vi "demod_table.vi"(2 "Light enables":bool[](array[boolean]), 3 "Block size":i32) -> (0 "Cosine table":dbl[][][](array[numeric]) format="%#.4f", 1 "Sine table":dbl[][][](array[numeric]) format="%#.4f")   [LabVIEW 2013]
uses:
  initialization/globals.vi
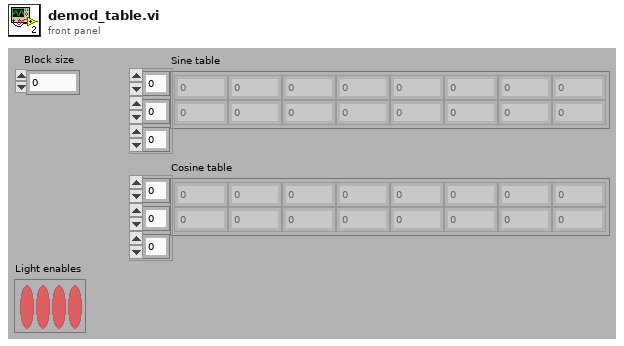
[diagram p1: front panel]
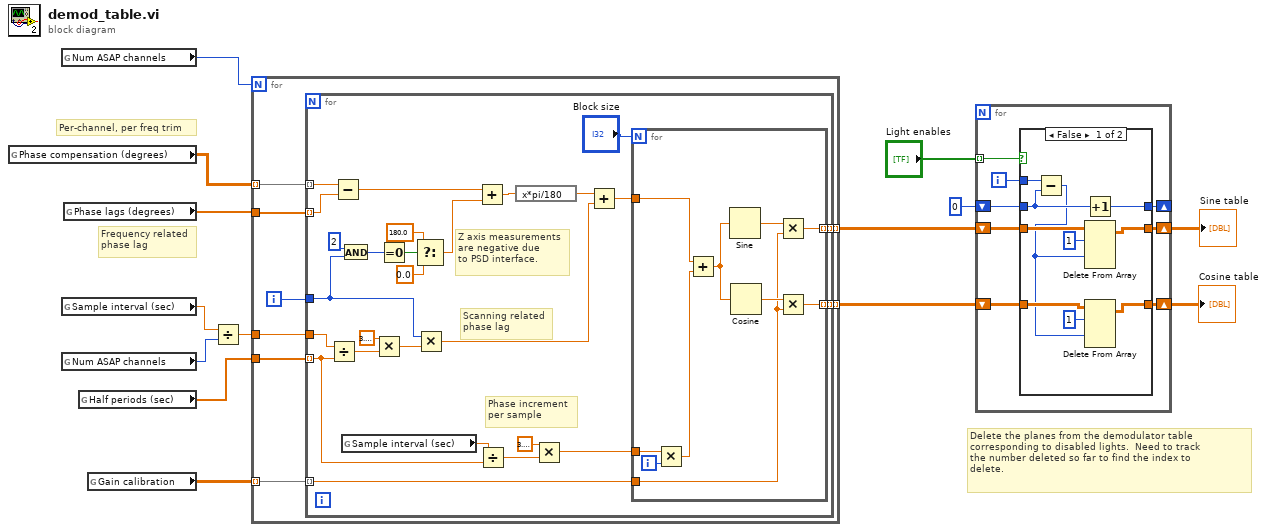
[diagram p0: block diagram]
diagram:
  # "Delete the planes from the demodulator table corresponding to disabled lights.  Need to track\nthe number deleted so far to find the index to\ndelete."
  # "Per-channel, per freq trim"
  # "Frequency related\nphase lag"
  n1 = global read "globals.vi" "Phase compensation (degrees)"() -> (w9:dbl[][])
  n2 = global read "globals.vi" "Num ASAP channels"() -> (w14:i32)
  n3 = global read "globals.vi" "Sample interval (sec)"() -> (w13:dbl)
  n4 = global read "globals.vi" "Num ASAP channels"() -> (w12:i32)
  n5 = global read "globals.vi" "Phase lags (degrees)"() -> (w8:dbl[])
  n6 = global read "globals.vi" "Half periods (sec)"() -> (w10:dbl[])
  n7 = global read "globals.vi" "Gain calibration"() -> (w1:sgl[][])
  n8 = Divide(x=w13, y=w12) -> (x/y=w11:dbl)
  n9 = for {
    N: w14 -> [_]
    tunnel: [w22] -> w7 mode=indexing
    tunnel: w11 -> [w21]
    tunnel: w8 -> [w19]
    tunnel: w10 -> [w18]
    tunnel: w9 -> [w17] mode=indexing
    tunnel: [w16] -> w6 mode=indexing
    tunnel: w1 -> [w15] mode=indexing
    i -> [w20]
    n10 = for {
      tunnel: [w49] -> w22 mode=indexing
      tunnel: w18 -> [w43] mode=indexing
      tunnel: w21 -> [w47]
      tunnel: w20 -> [w24]
      tunnel: w19 -> [w37] mode=indexing
      tunnel: w17 -> [w36] mode=indexing
      tunnel: [w35] -> w16 mode=indexing
      tunnel: w15 -> [w23] mode=indexing
      # "Z axis measurements\nare negative due\nto PSD interface."
      # "Phase increment\nper sample"
      # "Scanning related\nphase lag"
      n11 = Divide(x=w47, y=w43) -> (x/y=w46:dbl)
      n12 = Subtract(x=w36, y=w37) -> (x-y=w28:dbl)
      n13 = And(x=2 ("y"), y=w24) -> (x .and. y?=w34:i32)
      n14 = global read "globals.vi" "Sample interval (sec)"() -> (w44:dbl)
      n15 = Multiply(x=3.141592653589793, y=w46) -> (x*y=w26:dbl)
      n16 = Equal To 0?(x=w34) -> (x = 0?=w33:bool)
      n17 = Select(t=180.0, s=w33, f=0.0) -> (s? t:f=w29:dbl)
      n18 = Multiply(x=w24, y=w26) -> (x*y=w27:dbl)
      n19 = Add(x=w28, y=w29) -> (x+y=w30:dbl)
      n20 = Divide(x=w44, y=w43) -> (x/y=w41:dbl)
      n21 = expression code="x*pi/180"(w30) -> (w45:dbl)
      n22 = Multiply(x=3.141592653589793, y=w41) -> (x*y=w40:dbl)
      n23 = Add(x=w45, y=w27) -> (x+y=w39:dbl)
      n24 = for {
        N: "Block size" -> [_]
        tunnel: [w52] -> w49 mode=indexing
        tunnel: w40 -> [w58]
        tunnel: w39 -> [w57]
        tunnel: [w53] -> w35 mode=indexing
        tunnel: w23 -> [w50]
        i -> [w59]
        n25 = Multiply(x=w58, y=w59) -> (x*y=w56:dbl)
        n26 = Add(x=w57, y=w56) -> (x+y=w55:dbl)
        n27 = Sine(x=w55) -> (sin(x)=w51:dbl)
        n28 = Cosine(x=w55) -> (cos(x)=w54:dbl)
        n29 = Multiply(x=w51, y=w50) -> (x*y=w52:dbl)
        n30 = Multiply(x=w54, y=w50) -> (x*y=w53:dbl)
      }
    }
  }
  n31 = for {
    shift-right: [w65] -> w3
    shift-left: w7 -> [w66]
    shift-right: [w63] -> w4
    shift-left: w6 -> [w64]
    tunnel: "Light enables" -> [w67] mode=indexing
    shift-right: [w60] -> _
    shift-left: 0 -> [w61]
    i -> [w62]
    n32 = case shown="False" w67 {
      tunnel: w66 -> [w77 w80]
      tunnel: [w72 w80] -> w65
      tunnel: w64 -> [w74 w79]
      tunnel: [w73 w79] -> w63
      tunnel: w62 -> [w70 _]
      tunnel: w61 -> [w69 w78]
      tunnel: [w71 w78] -> w60
      frame False {
        n33 = Subtract(x=w70, y=w69) -> (x-y=w68:i32)
        n34 = Increment(x=w69) -> (x+1=w71:i32)
        n35 = Delete From Array(array=w77, length=1, index (dim 1)=w68) -> (array with subset deleted=w72:dbl[][][])  [unwired: 2 in, 1 out]
        n36 = Delete From Array(array=w74, length=1, index (dim 1)=w68) -> (array with subset deleted=w73:dbl[][][])  [unwired: 2 in, 1 out]
      }
      frame True {
      }
    }
  }
  "Sine table" <- w3
  "Cosine table" <- w4
